vi "DualCommWithProp.vi"() -> ()   [LabVIEW 2014]
uses:
  <vilib>/Instr/_visa.llb/VISA Configure Serial Port (Instr).vi
panel:
  out "Numeric":dbl
  out "str to byte":dbl[](array[numeric])
  in  "stop":bool
  out "Data":string
  in  "Rx from Prop Port":refnum<visa-resource-name>
  # "Dual Comm With Prop"
  # "Output from Prop:"
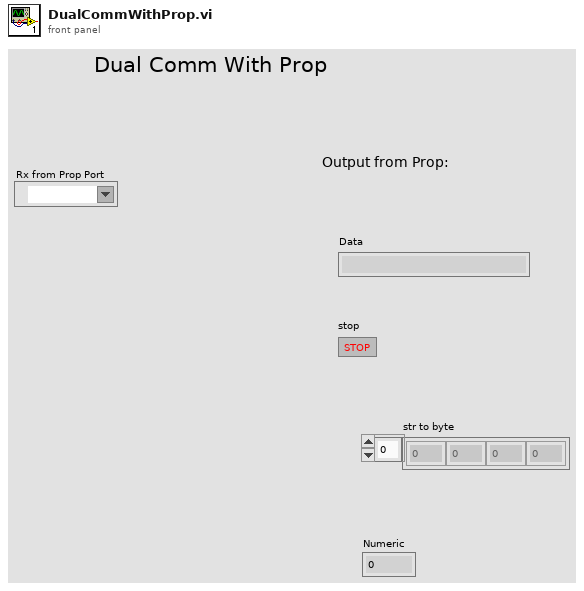
[diagram p1: front panel]
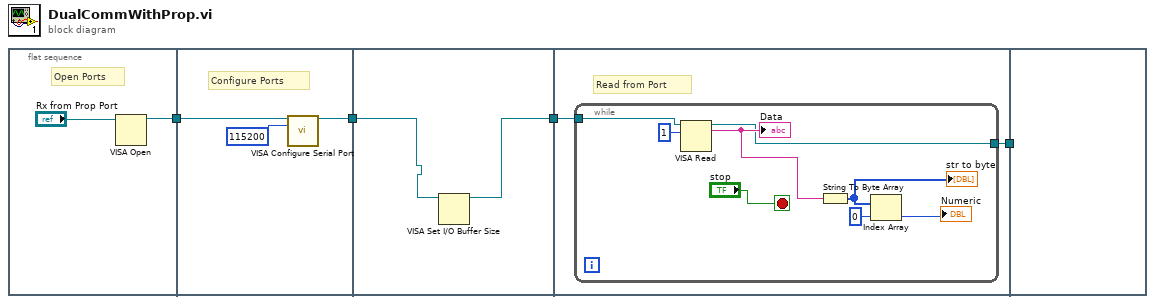
[diagram p0: block diagram]
diagram:
  n1 = flat-sequence {
    tunnel: [w5] -> w4
    tunnel: w4 -> [w9]
    tunnel: [w7] -> w3
    tunnel: w3 -> [w11]
    tunnel: [w10] -> w2
    tunnel: w2 -> [w13]
    tunnel: [w12] -> w1
    tunnel: w1 -> [_]
    frame #0 {
      # "Open Ports"
      n2 = VISA Open(VISA resource name="Rx from Prop Port") -> (VISA resource name=w5:refnum<visa-resource-name>)  [unwired: 4 in, 1 out]
    }
    frame #1 {
      # "Configure Ports"
      n3 = call-poly "VISA Configure Serial Port"("VISA resource name"=w9, "baud rate (9600)"=u32 115200) -> ("VISA resource name out"=w7:refnum<visa-resource-name>)  [unwired: 12 in, 1 out]
    }
    frame #2 {
      n4 = VISA Set I/O Buffer Size(VISA resource name=w11) -> (VISA resource name out=w10:refnum<visa-resource-name>)  [unwired: 3 in, 1 out]
    }
    frame #3 {
      # "Read from Port"
      n5 = while {
        tunnel: w13 -> [w15]
        tunnel: [w14] -> w12
        stop <- "stop" stop-if-true
        n6 = VISA Read(VISA resource name=w15, byte count=u32 1) -> (VISA resource name out=w14:refnum<visa-resource-name>, read buffer=w19:string)  [unwired: 1 in, 2 out]
        "Data" <- w19
        n7 = String To Byte Array(string=w19) -> (unsigned byte array=w17:u8[])
        "str to byte" <- w17
        n8 = Index Array(array=w17, index=0) -> (element=→"Numeric":u8)
      }
    }
    frame #4 {
    }
  }
